vi "Read Dev.Commands.vi"(8 "error in (no error)":errorcluster, 11 "SLSC Local in":refnum<class "SLSC Local.lvclass">) -> (0 "error out":errorcluster, 2 "Dev.Commands":refnum<k21>[](array[refnum]), 3 "SLSC Local out":refnum<class "SLSC Local.lvclass">)   [LabVIEW 2015, in "SLSC Local.lvclass"]
uses:
  SLSC Local.lvclass
  <resource>/objmgr/slsc.rc
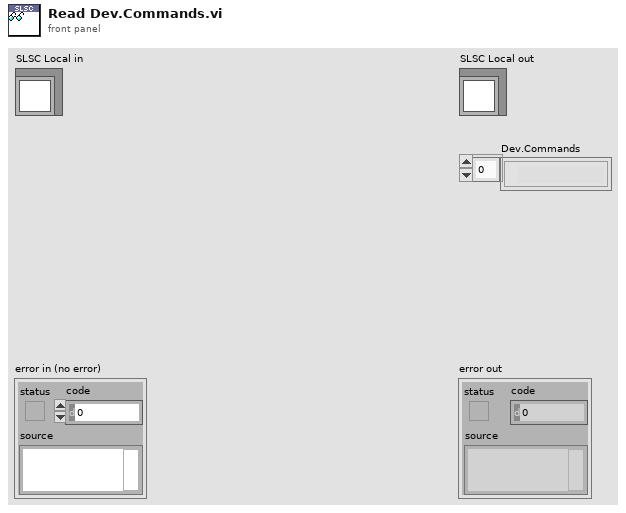
[diagram p1: front panel]
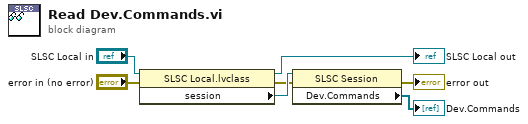
[diagram p0: block diagram]
diagram:
  n1 = property class="SLSC Local.lvclass"(reference="SLSC Local in", error in="error in (no error)") -> (reference out=→"SLSC Local out":refnum<class "SLSC Local.lvclass">, error out=w6:errorcluster, "session"=w7:refnum<k21>)
  n2 = property class="SLSC Session"(reference=w7, error in=w6) -> (error out=→"error out":errorcluster, "Dev.Commands"=→"Dev.Commands":refnum<k21>[])  [unwired: 1 out]
